vi "Measure_GetData.vi"(8 "error in (no error)":errorcluster, 9 "Variant":variant, 10 "SpectraCount":i32=1, 11 "Avantes in":refnum<class "Avantes.lvclass">) -> (0 "error out":errorcluster, 2 "Data_Raw":T1(array[cluster])=[{"Image"=array1x1x1410[1410 elements], "Frame Size"={"F"=0, "Y"=0, "X"=1410}}], 3 "Avantes out":refnum<class "Avantes.lvclass">, 5 "Time":dbl[](array[numeric])=[483691852.0])   [LabVIEW 2020, in "Avantes.lvclass"]
uses:
  <instrlib>/Classes/CCD/Avantes/Avantes.lvclass
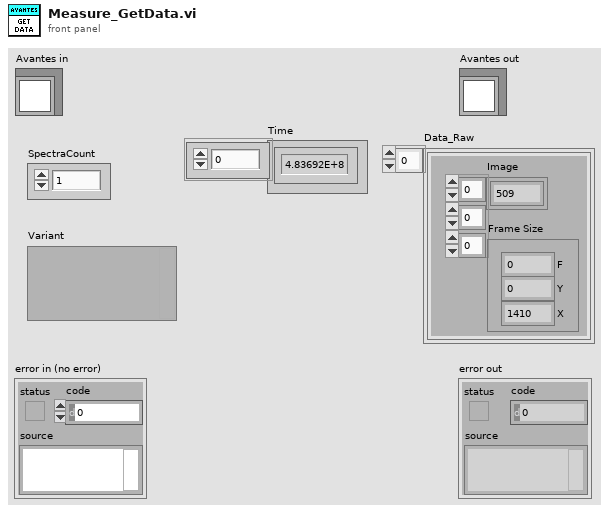
[diagram p1: front panel]
types:
  T1 = cluster{"Image":dbl[][][], "Frame Size":cluster{"F":i32, "Y":i32, "X":i32}}[]
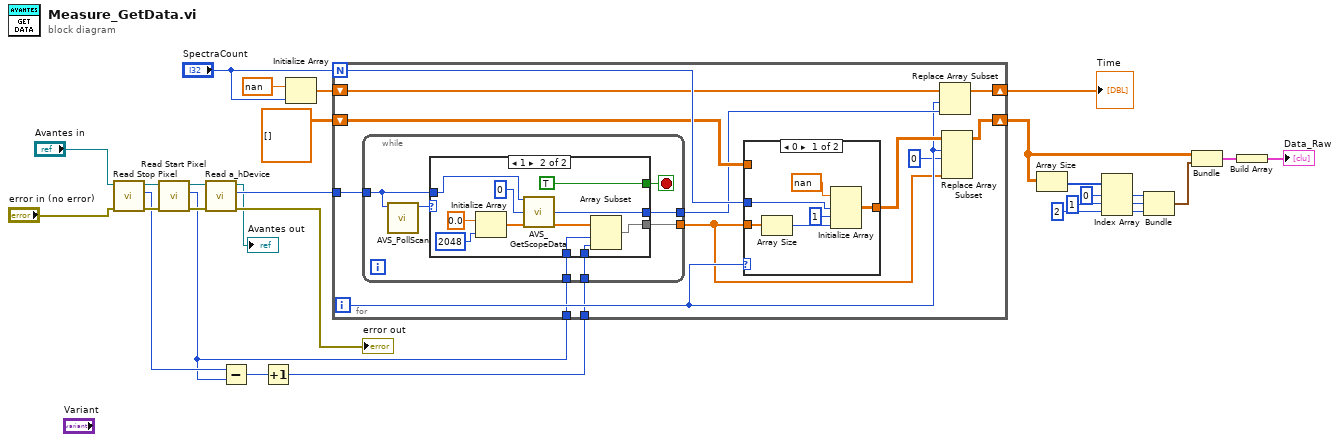
[diagram p0: block diagram]
diagram:
  n1 = call-dynamic "Read Stop Pixel.vi"("error in (no error)"="error in (no error)", "Avantes in"="Avantes in") -> ("error out"=w8:errorcluster, "Stop Pixel"=w2:u16, "Avantes out"=w7:refnum<class "Avantes.lvclass">)  [unwired: 7 in]
  n2 = call-dynamic "Read Start Pixel.vi"("error in (no error)"=w8, "Avantes in"=w7) -> ("error out"=w10:errorcluster, "Start Pixel"=w1:u16, "Avantes out"=w9:refnum<class "Avantes.lvclass">)  [unwired: 7 in]
  n3 = call-dynamic "Read a_hDevice.vi"("error in (no error)"=w10, "Avantes in"=w9) -> ("error out"=→"error out":errorcluster, "a_hDevice"=w29:i32, "Avantes out"=→"Avantes out":refnum<class "Avantes.lvclass">)  [unwired: 7 in]
  n4 = Subtract(x=w2, y=w1) -> (x-y=w4:u16)
  n5 = Increment(x=w4) -> (x+1=w3:u16)
  n6 = Initialize Array(nan ("element"), "SpectraCount") -> (w24:dbl[])
  n7 = for {
    N: "SpectraCount" -> [w41]
    tunnel: w29 -> [w42]
    shift-right: [w37] -> w22
    shift-left: w24 -> [w39]
    shift-right: [w35] -> w14
    shift-left: dbl[][][] [] -> [w40]
    tunnel: w1 -> [w31]
    tunnel: w3 -> [w30]
    i -> [w34]
    n8 = while {
      tunnel: w42 -> [w55]
      tunnel: [w53] -> w38
      tunnel: [w52] -> w32
      tunnel: w31 -> [w51]
      tunnel: w30 -> [w50]
      stop <- w54 stop-if-true
      n9 = call <instrlib>:"AVS_PollScan.vi"("a_hDevice"=w55) -> ("Output Value"=w56:i32)  [unwired: 8 in]
      n10 = case shown="1" w56 {
        tunnel: w55 -> [_ w64]
        tunnel: [_ TRUE] -> w54
        tunnel: [_ w62] -> w53
        tunnel: [_ w57] -> w52
        tunnel: w51 -> [_ w59]
        tunnel: w50 -> [_ w58]
        frame 0, Default {
        }
        frame 1 {
          n11 = Initialize Array(0.0 ("element"), 2048 ("dimension size")) -> (w66:dbl[])
          n12 = call <instrlib>:"AVS_GetScopeData.vi"("a_hDevice"=w64, "a_pTimeLabel"=u32 0, "a_pSpectrum"=w66) -> ("a_pTimeLabel"=w62:u32, "a_pSpectrum"=w60:dbl[])  [unwired: 10 in, 1 out]
          n13 = Array Subset(array=w60, index=w59, length=w58) -> (w57:dbl[])
        }
      }
    }
    n14 = case shown="0" w34 {
      tunnel: w32 -> [w47 _]
      tunnel: w41 -> [w44 _]
      tunnel: [w43 w49] -> w36
      tunnel: w40 -> [_ w49]
      frame 0 {
        n15 = Array Size(array=w47) -> (size(s)=w46:i32)
        n16 = Initialize Array(nan ("element"), w44, 1 ("dimension size"), w46) -> (w43:dbl[][][])
      }
      frame Default {
      }
    }
    n17 = Replace Array Subset(array=w39, new element=w38, index=w34) -> (w37:dbl[])
    n18 = Replace Array Subset(array=w36, new element=w32, index (dim 0)=w34, index (dim 1)=0 ("disabled index (row)")) -> (w35:dbl[][][])  [unwired: 1 in]
  }
  "Time" <- w22
  n19 = Array Size(array=w14) -> (size(s)=w21:i32[])
  n20 = Index Array(array=w21, index #1=0 ("index"), index #2=1 ("index"), index #3=2 ("index")) -> (element #1=w17:i32, element #2=w16:i32, element #3=w15:i32)
  n21 = Bundle(w17, w16, w15) -> (w28:cluster{i32, i32, i32})  [unwired: 1 in]
  n22 = Bundle(w14, w28) -> (w13:cluster{dbl[][][], cluster{i32, i32, i32}})  [unwired: 1 in]
  n23 = Build Array(w13) -> (→"Data_Raw":cluster{dbl[][][], cluster{i32, i32, i32}}[])
